vi "D2SParser - Private - Function - Read CRC.vi"(8 "error in (no error)":errorcluster, 11 "D2SParser in":refnum<class "D2SParser.lvclass">) -> (0 "error out":errorcluster, 3 "D2SParser out":refnum<class "D2SParser.lvclass">)   [LabVIEW 2015, in "D2SParser.lvclass"]
uses:
  D2SParser.lvclass
  D2SParser.lvclass/D2SParser.ctl
  D2SParser - Private - Helper - Read Long.vi
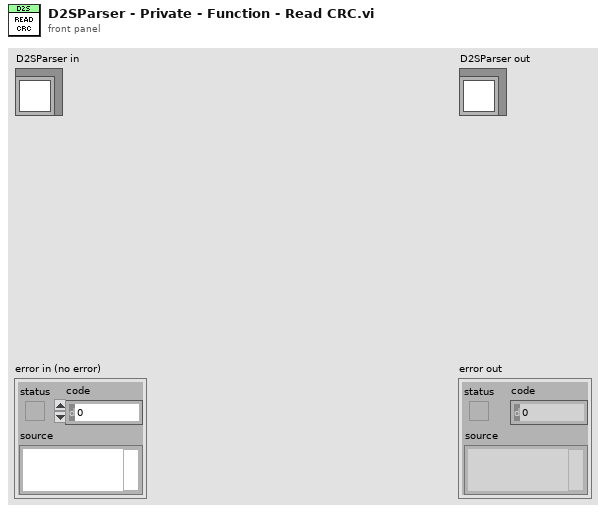
[diagram p1: front panel]
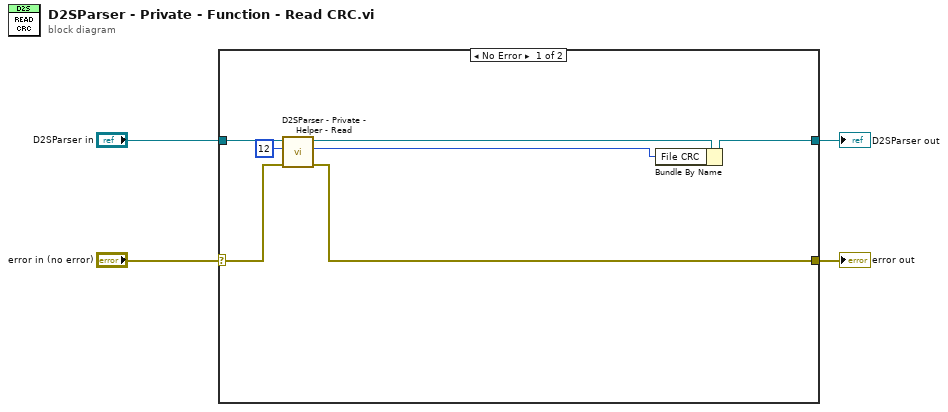
[diagram p0: block diagram]
diagram:
  n1 = case shown="No Error" "error in (no error)" {
    selector: "error in (no error)" -> [w10 w13]
    tunnel: [w8 w13] -> w3
    tunnel: [w6 w12] -> w1
    tunnel: "D2SParser in" -> [w11 w12]
    frame No Error {
      n2 = call-poly "D2SParser - Private - Helper - Read.vi"("error in (no error)"=w10, "Position"=i64 12, "D2SParser in"=w11) -> ("error out"=w8:errorcluster, "long"=w5:u32, "D2SParser out"=w9:refnum<class "D2SParser.lvclass">)  [unwired: 6 in]
      n3 = Bundle By Name(cluster=w9, "File CRC"=w5) -> (w6:refnum<class "D2SParser.lvclass">)
    }
    frame Error {
    }
  }
  "error out" <- w3
  "D2SParser out" <- w1
